vi "writeSaveData.vi"(8 "error in (no error)":errorcluster, 11 "reference in":refnum<class "excelFile.lvclass">) -> (0 "error out":errorcluster, 3 "reference out":refnum<class "excelFile.lvclass">)   [LabVIEW 2015, in "excelFile.lvclass"]
uses:
  excelFile.lvclass
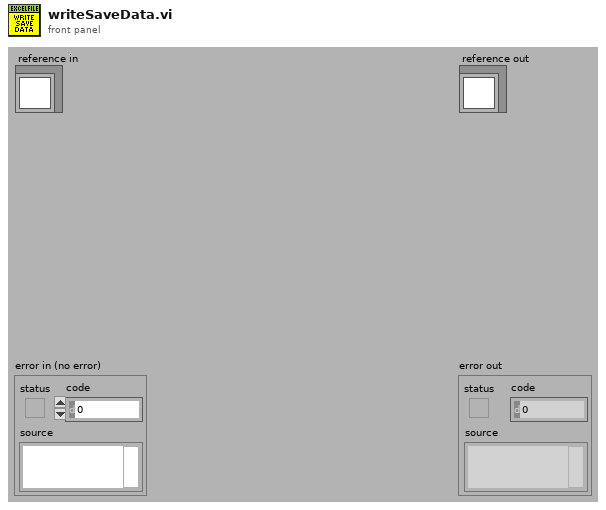
[diagram p1: front panel]
types:
  T1 = typedef "excelFile.lvclass/ObjectAttributesRef.ctl" = refnum<data-value>
  T2 = typedef "excelFile.lvclass/ObjectAttributes.ctl" = cluster{"MyAttribute":dbl, "path":string, "Refnum Excel":cluster{"Excel._Application":refnum<k7>, "Workbooks":refnum<k7>, "Open":refnum<k7>}, "data":string[][][], "fileType":T3, "sheetName":string[]}
  T3 = typedef "excelFile.lvclass/fileType.ctl" = enum16{"database", "CosmedTest PFTSUITE", "CosmedTest OMNIA"}
  T4 = cluster{"Excel._Application":refnum<k7>, "Workbooks":refnum<k7>, "Open":refnum<k7>}
  T5 = cluster{"Excel._Application":refnum<k7>, "Workbooks":refnum<k7>, "Open":refnum<k7>, "Worksheets":refnum<k7>, "Excel._Worksheet":refnum<k7>}
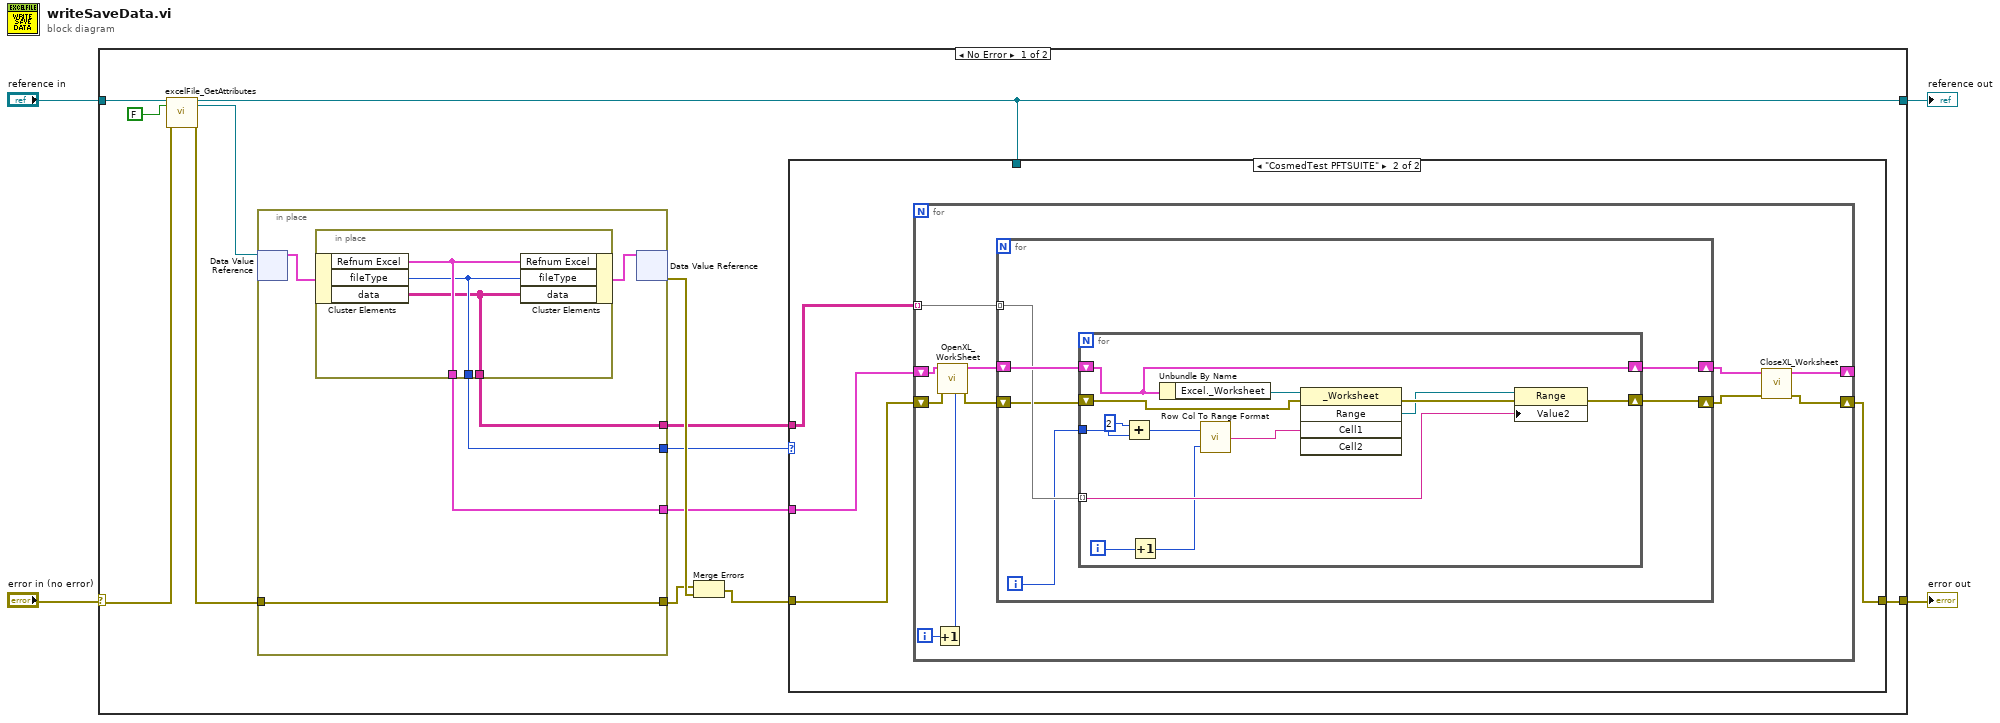
[diagram p0: block diagram]
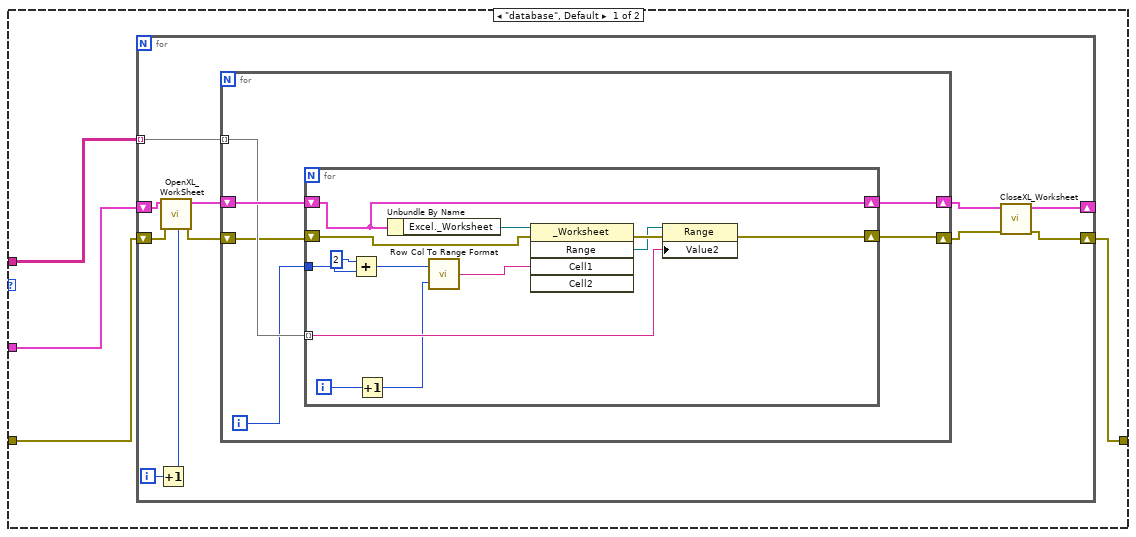
[diagram p2: hidden frame]
diagram:
  n1 = case shown="No Error" "error in (no error)" {
    selector: "error in (no error)" -> [w13 w96]
    tunnel: [w9 w96] -> w3
    tunnel: [w8 w95] -> w1
    tunnel: "reference in" -> [w15 w95]
    frame No Error {
      n2 = call "excelFile_GetAttributes.vi"("reference in"=w15, "return data? (T)"=FALSE, "error in (no error)"=w13) -> ("reference out"=w8:refnum<class "excelFile.lvclass">, "attributes ref"=w11:T1, "error out"=w12:errorcluster)  [unwired: 13 in, 1 out]
      n3 = in-place {
        in-place-border: w12 -> [w89]
        in-place-border: [w89] -> w16
        in-place-border: [w88] -> w7
        in-place-border: [w87] -> w6
        in-place-border: [w86] -> w5
        n4 = in-place-dvr #1(w11) -> (w90:T2)  [unwired: 1 out]
        n5 = in-place {
          in-place-border: [w94] -> w88
          in-place-border: [w93] -> w87
          in-place-border: [w92] -> w86
          n6 = in-place-cluster #2(w90) -> ("Refnum Excel"=w94:T4, "fileType"=w93:T3, "data"=w92:string[][][])
          n7 = in-place-cluster #2("Refnum Excel"=w94, "fileType"=w93, "data"=w92) -> (w91:T2)
        }
        n8 = in-place-dvr #1(w91) -> (w17:errorcluster)  [unwired: 1 out]
      }
      n9 = Merge Errors(w16, w17) -> (w10:errorcluster)
      n10 = case shown="\"CosmedTest PFTSUITE\"" w6 {
        tunnel: w10 -> [w19 w53]
        tunnel: [w18 w52] -> w9
        tunnel: w7 -> [w21 w54]
        tunnel: w8 -> [_ _]
        tunnel: w5 -> [w20 w55]
        frame "database", Default {
          n11 = for {
            tunnel: w20 -> [w32] mode=indexing
            shift-right: [w25] -> w18
            shift-left: w19 -> [w29]
            shift-right: [w24] -> _
            shift-left: w21 -> [w23]
            i -> [w30]
            n12 = Increment(x=w30) -> (x+1=w22:i32)
            n13 = call <userlib>:"OpenXL_WorkSheet.vi"("Sheet"=w22, "error in (no error)"=w29, "Refnum Cluster In"=w23) -> ("error out"=w28:errorcluster, "Refnum Cluster Out"=w31:T5)  [unwired: 7 in]
            n14 = for {
              tunnel: w32 -> [w37] mode=indexing
              shift-right: [w35] -> w27
              shift-left: w31 -> [w38]
              shift-right: [w34] -> w26
              shift-left: w28 -> [w33]
              i -> [w36]
              n15 = for {
                tunnel: w37 -> [w47] mode=indexing
                tunnel: w36 -> [w45]
                shift-right: [w44] -> w35
                shift-left: w38 -> [w44]
                shift-right: [w43] -> w34
                shift-left: w33 -> [w42]
                i -> [w46]
                n16 = Add(x=2, y=w45) -> (x+y=w41:i32)
                n17 = Increment(x=w46) -> (x+1=w40:i32)
                n18 = Unbundle By Name(w44) -> ("Excel._Worksheet"=w51:refnum<k7>)
                n19 = call <userlib>:"Row Col To Range Format.vi"("Column"=w40, "Row"=w41) -> ("Output String"=w50:string)
                n20 = invoke class="_Worksheet" method="Range"(reference=w51, error in=w42, "Cell1"=w50) -> (error out=w49:errorcluster, "Range"=w48:refnum<k7>)  [unwired: 2 in, 3 out]
                n21 = property class="Range"(reference=w48, error in=w49, "Value2"=w47) -> (error out=w43:errorcluster)  [unwired: 1 out]
              }
            }
            n22 = call <userlib>:"CloseXL_Worksheet.vi"("error in (no error)"=w26, "Refnum Cluster In"=w27) -> ("error out"=w25:errorcluster, "Refnum Cluster Out"=w24:T4)  [unwired: 8 in]
          }
        }
        frame "CosmedTest PFTSUITE" {
          n23 = for {
            tunnel: w55 -> [w66] mode=indexing
            shift-right: [w59] -> w52
            shift-left: w53 -> [w63]
            shift-right: [w58] -> _
            shift-left: w54 -> [w57]
            i -> [w64]
            n24 = Increment(x=w64) -> (x+1=w56:i32)
            n25 = call <userlib>:"OpenXL_WorkSheet.vi"("Sheet"=w56, "error in (no error)"=w63, "Refnum Cluster In"=w57) -> ("error out"=w62:errorcluster, "Refnum Cluster Out"=w65:T5)  [unwired: 7 in]
            n26 = for {
              tunnel: w66 -> [w71] mode=indexing
              shift-right: [w69] -> w61
              shift-left: w65 -> [w72]
              shift-right: [w68] -> w60
              shift-left: w62 -> [w67]
              i -> [w70]
              n27 = for {
                tunnel: w71 -> [w82] mode=indexing
                tunnel: w70 -> [w80]
                shift-right: [w79] -> w69
                shift-left: w72 -> [w79]
                shift-right: [w78] -> w68
                shift-left: w67 -> [w77]
                i -> [w81]
                n28 = Add(x=2, y=w80) -> (x+y=w76:i32)
                n29 = Increment(x=w81) -> (x+1=w75:i32)
                n30 = Unbundle By Name(w79) -> ("Excel._Worksheet"=w73:refnum<k7>)
                n31 = call <userlib>:"Row Col To Range Format.vi"("Column"=w75, "Row"=w76) -> ("Output String"=w85:string)
                n32 = invoke class="_Worksheet" method="Range"(reference=w73, error in=w77, "Cell1"=w85) -> (error out=w84:errorcluster, "Range"=w83:refnum<k7>)  [unwired: 2 in, 3 out]
                n33 = property class="Range"(reference=w83, error in=w84, "Value2"=w82) -> (error out=w78:errorcluster)  [unwired: 1 out]
              }
            }
            n34 = call <userlib>:"CloseXL_Worksheet.vi"("error in (no error)"=w60, "Refnum Cluster In"=w61) -> ("error out"=w59:errorcluster, "Refnum Cluster Out"=w58:T4)  [unwired: 8 in]
          }
        }
      }
    }
    frame Error {
    }
  }
  "error out" <- w3
  "reference out" <- w1
